vi "Write DC Offset Cluster.vi"(8 "error in (no error)":errorcluster, 10 "DC Offset Cluster":T1, 11 "Device in":refnum<class "Device.lvclass">) -> (0 "error out":errorcluster, 3 "Device out":refnum<class "Device.lvclass">)   [LabVIEW 2020, in "Device.lvclass"]
uses:
  Device.lvclass
  Controls/DC Offset Cluster.ctl
  Instruments/Power Supply/Power Supply.lvclass
  Device.lvclass/Device.ctl
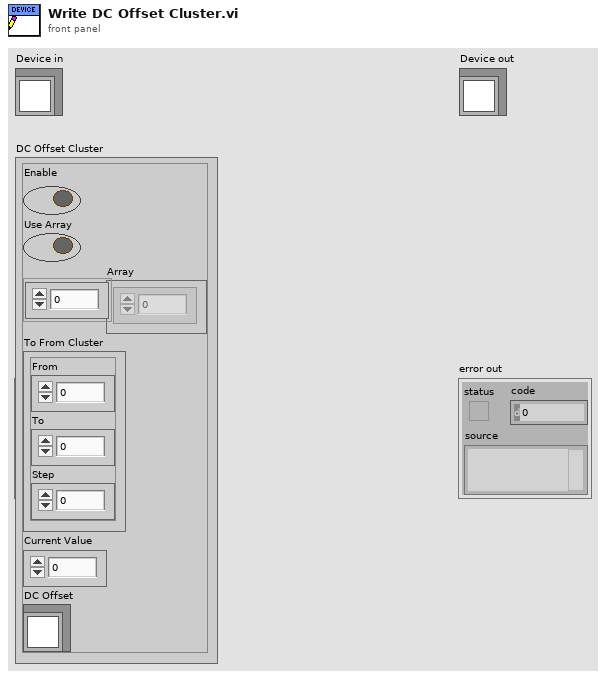
[diagram p1: front panel]
types:
  T1 = typedef "Device.lvclass/DC Offset Cluster.ctl" = cluster{"Enable":bool, "Use Array":bool, "Array":dbl[], "To From Cluster":cluster{"From":dbl, "To":dbl, "Step":dbl}, "Current Value":dbl, "DC Offset":refnum<class "Power Supply.lvclass">}
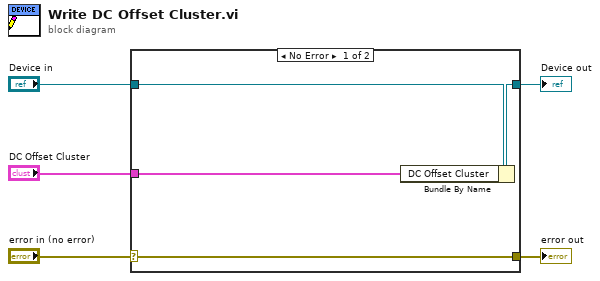
[diagram p0: block diagram]
diagram:
  n1 = case shown="No Error" "error in (no error)" {
    selector: "error in (no error)" -> [w9 w10]
    tunnel: [w9 w10] -> w4
    tunnel: [w7 w11] -> w2
    tunnel: "Device in" -> [w8 w11]
    tunnel: "DC Offset Cluster" -> [w6 _]
    frame No Error {
      n2 = Bundle By Name(cluster=w8, "DC Offset Cluster"=w6) -> (w7:refnum<class "Device.lvclass">)
    }
    frame Error {
    }
  }
  "error out" <- w4
  "Device out" <- w2
